vi "ELRecvReady.vi"() -> (0 "connection ID":refnum<k16>)   [LabVIEW 2017]
uses:
  <vilib>/Utility/tcp.llb/UDP Multicast Read-Only Open.vi
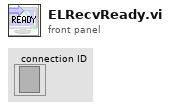
[diagram p1: front panel]
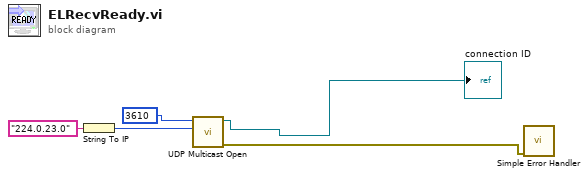
[diagram p0: block diagram]
diagram:
  n1 = String To IP(1:"224.0.23.0") -> (0:w4:u32)
  n2 = call-poly <vilib>:"UDP Multicast Open.vi"("multicast addr"=w4, "port"=3610) -> ("error out"=w1:errorcluster, "connection ID"=→"connection ID":refnum<k16>)  [unwired: 7 in, 1 out]
  n3 = call <vilib>:"Simple Error Handler.vi"("error in (no error)"=w1) -> ()  [unwired: 4 in, 5 out]
